vi "Arm Actuator Controller.vi"(8 "error in":errorcluster) -> ()   [LabVIEW 2017]
doc: "This VI executes continuously carrying out the current operation and responding to updates or new operations. It will often contain the timing or control code that is difficult to place directly in TeleOp. This VI generally opens all sensors and motors and isolates the rest of the robot code from knowing how the operations are carried out."
uses:
  <vilib>/Rock Robotics/WPI/Framework/Completion Status.ctl
  Arm Actuator Setpoints.ctl
  Arm Actuator Operations.ctl
  Users/Public/Documents/Cross The Road Electronics/Phoenix-LabVIEW/Motor Controller/Controls/CTRE_Phoenix_MotorControl_ControlMode.ctl
  <vilib>/Rock Robotics/WPI/ThirdParty/Phoenix-LabVIEW/Motor Controller/Controls/CTRE_Phoenix_MotorControl_NeutralMode.ctl
  <vilib>/Rock Robotics/WPI/Solenoid/WPI_SolenoidValue.ctl
  <vilib>/Rock Robotics/WPI/Solenoid/WPI_SolenoidChannel.ctl
  <vilib>/Rock Robotics/WPI/Solenoid/WPI_SolenoidSetEnum.vi
  <vilib>/Rock Robotics/WPI/Solenoid/WPI_SolenoidOpenSingle.vi
  <vilib>/Rock Robotics/Network Tables/NT Write Boolean.vi
panel:
  in  "Interactive Values":T1
  out "Current\nCmd":string
  in  "Buttons":cluster{"Execute Cmd":bool, "Abort Cmd":bool}
  out "Command Timing":cluster{"Start Time (ms)":u32, "Iterations":i32}
  out "Status":T3
  # "Tip: It may be helpful to observe inputs and sensor values.\nYou may also want to display tuning or debugging controls."
  # "Interactive Command: You may fill in the settings for a command\nand schedule it with the Execute button. You can observe and abort\nany command while fine tuning the code for the controller."
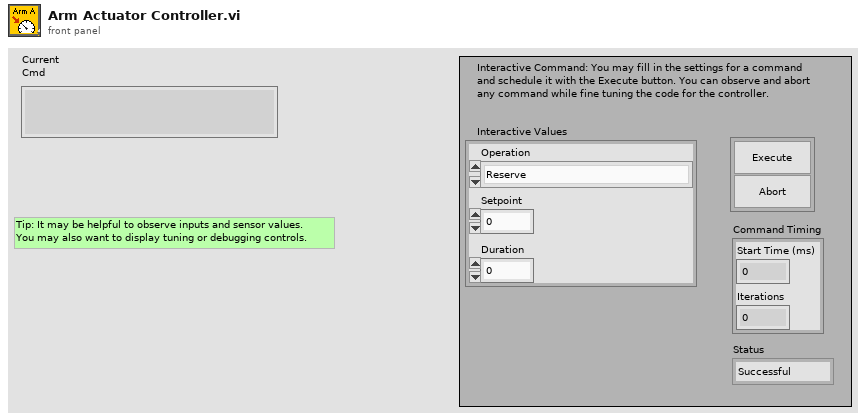
[diagram p1: front panel]
types:
  T1 = typedef "Arm Actuator Setpoints.ctl" = cluster{"Operation":T2, "Setpoint":dbl, "Duration":dbl}
  T2 = typedef "Arm Actuator Operations.ctl" = enum16{"Reserve", "Read Current", "Immediate", "Move Arm", "Claw In", "Claw Out"}
  T3 = typedef "Completion Status.ctl" = enum16{"Successful", "Aborted", "Incomplete"}
  T4 = typedef "WPI_SolenoidChannel.ctl" = enum8{"Solenoid 0", "Solenoid 1", "Solenoid 2", "Solenoid 3", "Solenoid 4", "Solenoid 5", "Solenoid 6", "Solenoid 7", "Invalid"}
  T5 = typedef "WPI_SolenoidValue.ctl" = enum16{"Off", "On", "Forward", "Reverse"}
  T6 = typedef "CTRE_Phoenix_MotorControl_NeutralMode.ctl" = enum8{"EEPROMSetting", "Override to Coast", "Override to Brake"}
  T7 = typedef "CTRE_Phoenix_MotorControl_ControlMode.ctl" = u16
  T8 = typedef "WPI_SolenoidDevRef.ctl" = cluster{"DevStatus":errorcluster, "Pneumatics Control Module":u8, "Forward Solenoid Channel":T4, "Reverse Solenoid Channel":T4}
  T9 = typedef "WPI_MotorControlDeviceRef.ctl" = cluster{"DeviceStatus":errorcluster, "Type":T10, "PWM":cluster{"PWM Channel":T11, "DeadBand":T12}, "CAN":cluster{"Device Number":u8, "SetOutput VI Ref":variant, "GetOutput VI Ref":variant, "Enable VI Ref":variant, "Disable VI Ref":variant, "Data":variant}, "Invert":bool, "DIO PWM":cluster{"PWM \"Enable\" Channel":T11, "DIOChannel":T13, "PWM Rate":dbl}}
  T10 = typedef "WPI_MotorControlType.ctl" = enum16{"PWM", "CAN", "DIO PWM"}
  T11 = typedef "FPGA_DIOPWMChannel.ctl" = enum8{"PWM 0", "PWM 1", "PWM 2", "PWM 3", "PWM 4", "PWM 5", "PWM 6", "PWM 7", "PWM 8", "PWM 9", "PWM MXP 0", "PWM MXP 1", "PWM MXP 2", "PWM MXP 3", "PWM MXP 4", "PWM MXP 5", "PWM MXP 6", "PWM MXP 7", "PWM MXP 8", "PWM MXP 9", "Invalid"}
  T12 = typedef "WPI_PWMDeadband.ctl" = cluster{"Name":string, "maxPositivePwm":i32, "minPositivePwm":i32, "centerPwm":i32, "maxNegativePwm":i32, "minNegativePwm":i32, "angularRange":u16}
  T13 = typedef "FPGA_DIOChannel.ctl" = enum8{"DIO 0", "DIO 1", "DIO 2", "DIO 3", "DIO 4", "DIO 5", "DIO 6", "DIO 7", "DIO 8", "DIO 9", "DIO MXP 0", "DIO MXP 1", "DIO MXP 2", "DIO MXP 3", "DIO MXP 4", "DIO MXP 5", "DIO MXP 6", "DIO MXP 7", "DIO MXP 8", "DIO MXP 9", "DIO MXP 10", "DIO MXP 11", "DIO MXP 12", "DIO MXP 13", "DIO MXP 14", "DIO MXP 15", "SPI Port CS1", "SPI Port CS2", "SPI Port CS3", "SPI Port MISO", "SPI Port MOSI", "Invalid"}
  T14 = typedef "Command Status Info.ctl" = cluster{"Name":string, "Status":T3, "notifier out":T15}
  T15 = typedef "Completion Notifier.ctl" = refnum<notifier>
  T16 = cluster{"Current Command":T1, "Command Timing":cluster{"Start Time (ms)":u32, "Iterations":i32}, "Command Arguments":cluster{"Command Info":T14, "Description":string, "Default Command":T1, "queue out":refnum<queue>, "Subsystem Name":string}}
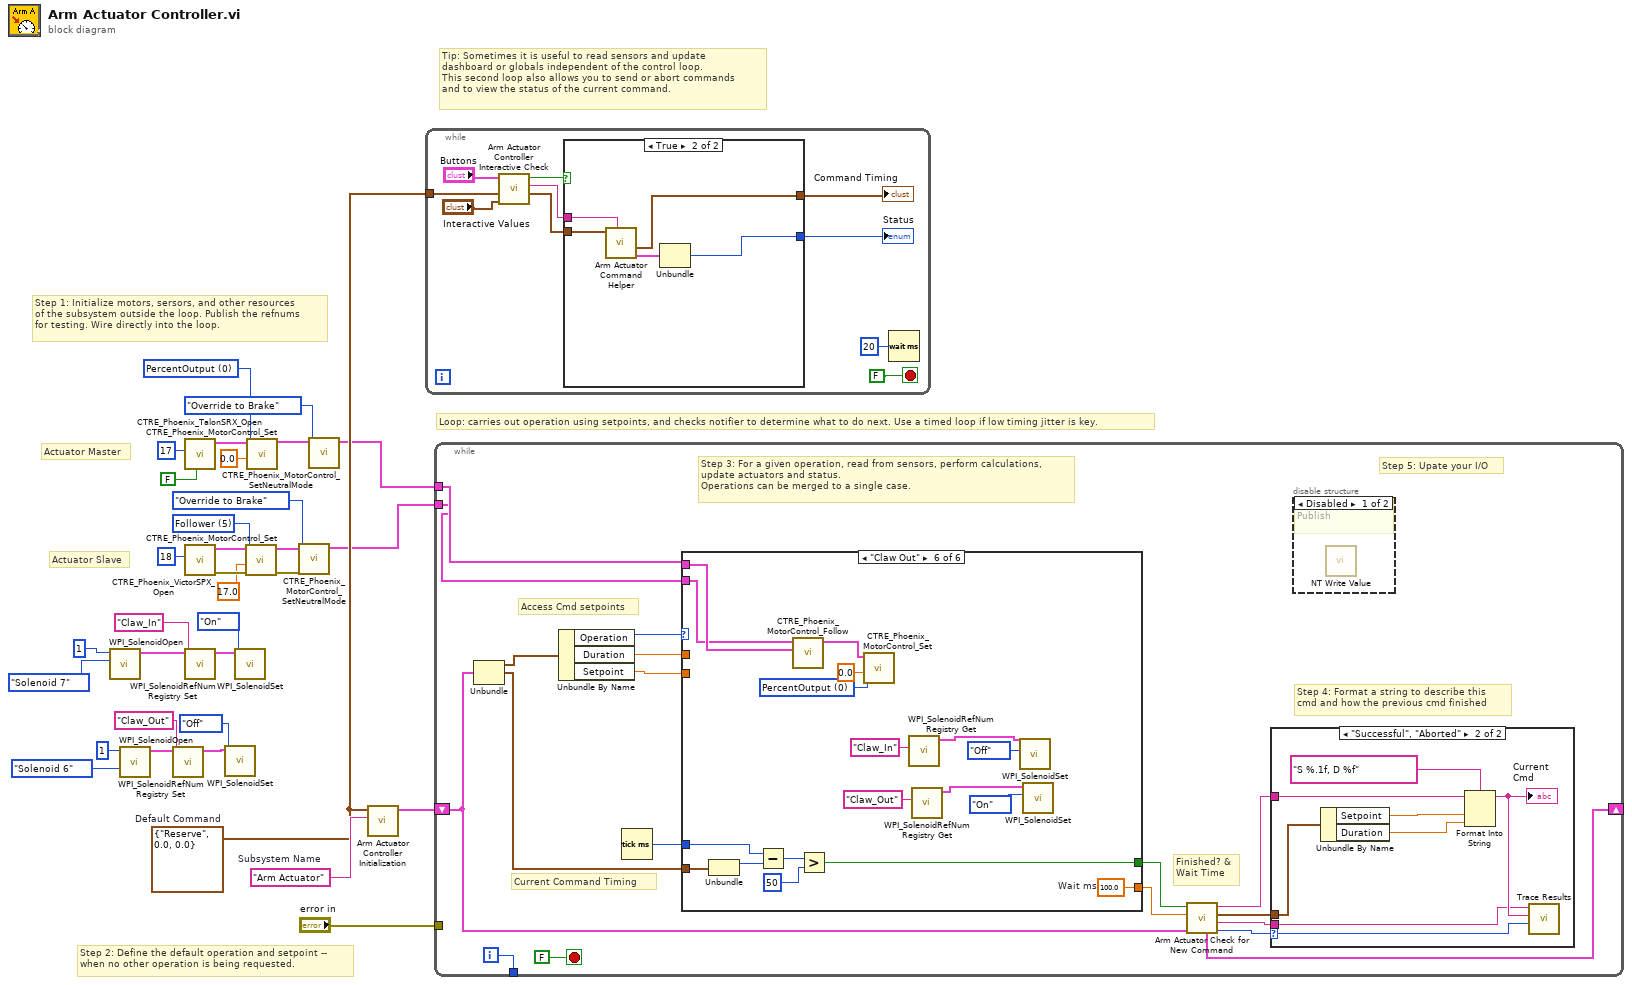
[diagram p0: block diagram]
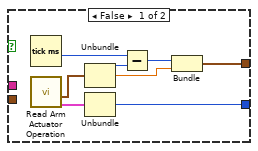
[diagram p2: hidden frame]
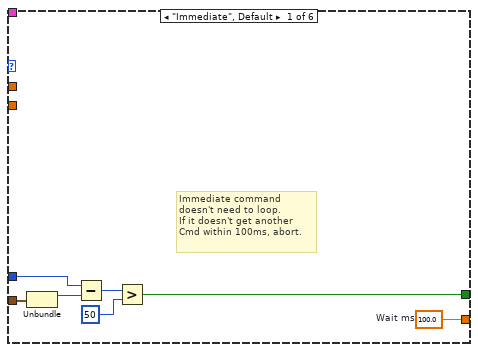
[diagram p5: hidden frame]
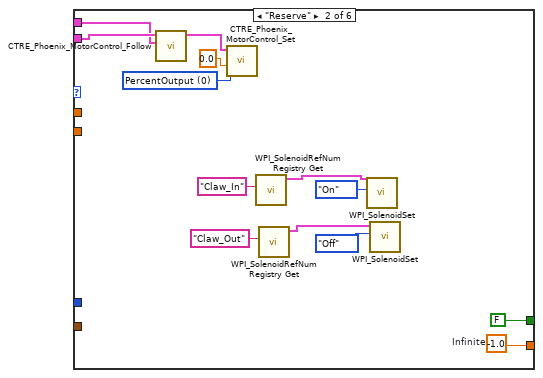
[diagram p6: hidden frame]
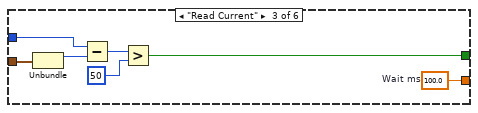
[diagram p7: hidden frame]
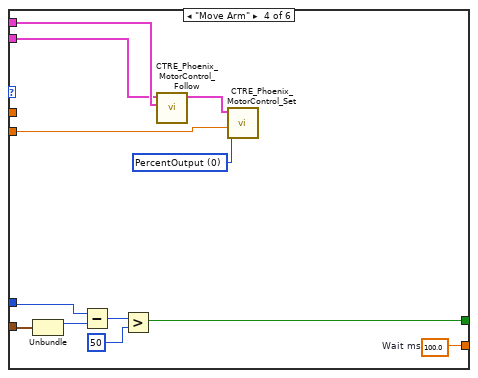
[diagram p8: hidden frame]
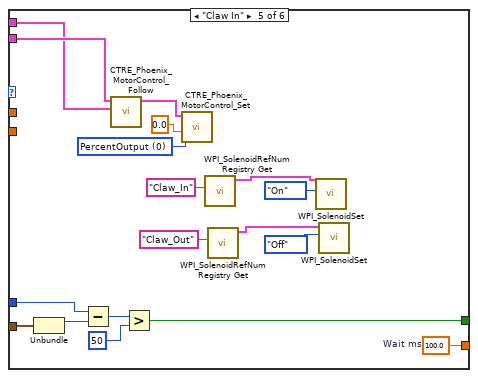
[diagram p9: hidden frame]
diagram:
  w15 = T7 5 items=["PercentOutput"=0, "Position"=1, "Velocity"=2, "Current"=3, "Follower"=5, "MotionProfile"=6, "MotionMagic"=7, "MotionMagicArc"=8, "MotionProfileArc"=10, "Disabled"=15] ("Control Mode")
  w22 = T7 0 items=["PercentOutput"=0, "Position"=1, "Velocity"=2, "Current"=3, "Follower"=5, "MotionProfile"=6, "MotionMagic"=7, "MotionMagicArc"=8, "MotionProfileArc"=10, "Disabled"=15] ("Control Mode")
  w30 = T1 {"Operation"=enum."Reserve", "Setpoint"=0.0, "Duration"=0.0}  # Default Command
  w31 = "Arm Actuator"  # Subsystem Name
  # "Actuator Slave"
  # "Actuator Master"
  # "Tip: Sometimes it is useful to read sensors and update\ndashboard or globals independent of the control loop.\nThis second loop also allows you to send or abort commands\nand to view the status of the current command."
  # "Step 2: Define the default operation and setpoint --\nwhen no other operation is being requested."
  # "Step 1: Initialize motors, sersors, and other resources\nof the subsystem outside the loop. Publish the refnums\nfor testing. Wire directly into the loop."
  # "Loop: carries out operation using setpoints, and checks notifier to determine what to do next. Use a timed loop if low timing jitter is key."
  n1 = call-poly <vilib>:"WPI_SolenoidOpen.vi"("Solenoid Channel"=WPI_SolenoidChannel."Solenoid 7", "Pneumatics Control Module (0)"=u8 1) -> ("SolenoidDevRef"=w29:T8)  [unwired: 8 in, 1 out]
  n2 = call-poly <vilib>:"WPI_SolenoidOpen.vi"("Solenoid Channel"=WPI_SolenoidChannel."Solenoid 6", "Pneumatics Control Module (0)"=u8 1) -> ("SolenoidDevRef"=w27:T8)  [unwired: 8 in, 1 out]
  n3 = call <vilib>:"WPI_SolenoidRefNum Registry Set.vi"("refnum name"="Claw_Out", "SolenoidDevRef"=w27) -> ("SolenoidDevRef"=w8:T8)  [unwired: 8 in, 1 out]
  n4 = call <vilib>:"CTRE_Phoenix_TalonSRX_Open.vi"("Invert"=FALSE, "Device Number"=u8 17) -> ("CAN Talon SRX Ref"=w23:T9)  [unwired: 8 in, 1 out]
  n5 = call <vilib>:"CTRE_Phoenix_VictorSPX_Open.vi"("Device Number"=u8 18) -> ("error out"=w17:errorcluster, "CAN Talon SRX Ref"=w16:T9)  [unwired: 9 in]
  n6 = call <vilib>:"WPI_SolenoidRefNum Registry Set.vi"("refnum name"="Claw_In", "SolenoidDevRef"=w29) -> ("SolenoidDevRef"=w6:T8)  [unwired: 8 in, 1 out]
  n7 = call-poly <vilib>:"WPI_SolenoidSet.vi"("Value"=WPI_SolenoidValue."Off", "SolenoidDevRef"=w8) -> ()  [unwired: 8 in, 2 out]
  n8 = call-poly <vilib>:"WPI_SolenoidSet.vi"("Value"=WPI_SolenoidValue."On", "SolenoidDevRef"=w6) -> ()  [unwired: 8 in, 2 out]
  n9 = call <vilib>:"CTRE_Phoenix_MotorControl_Set.vi"("error in (no error)"=w17, "Output"=17.0, "Control Mode"=w15, "PhoenixMotorControlDevRef"=w16) -> ("error out"=w13:errorcluster, "PhoenixMotorControlDevRef"=w12:T9)  [unwired: 6 in]
  n10 = call <vilib>:"CTRE_Phoenix_MotorControl_Set.vi"("Output"=0.0, "Control Mode"=w22, "PhoenixMotorControlDevRef"=w23) -> ("PhoenixMotorControlDevRef"=w20:T9)  [unwired: 7 in, 1 out]
  n11 = call <vilib>:"CTRE_Phoenix_MotorControl_SetNeutralMode.vi"("error in (no error)"=w13, "Motor Control Neutral Mode"=CTRE_Phoenix_MotorControl_NeutralMode."Override to Brake", "PhoenixMotorControlDevRef"=w12) -> ("PhoenixMotorControlDevRef"=w9:T9)  [unwired: 7 in, 1 out]
  n12 = call <vilib>:"CTRE_Phoenix_MotorControl_SetNeutralMode.vi"("Motor Control Neutral Mode"=CTRE_Phoenix_MotorControl_NeutralMode."Override to Brake", "PhoenixMotorControlDevRef"=w20) -> ("PhoenixMotorControlDevRef"=w10:T9)  [unwired: 8 in, 1 out]
  n13 = call "Arm Actuator Controller Initialization.vi"("Subsystem Name"=w31, "Default Command"=w30) -> ("Current Command"=w32:T16)  [unwired: 9 in]
  n14 = while {
    tunnel: w30 -> [w40]
    stop <- FALSE stop-if-true
    n15 = call "Arm Actuator Controller Interactive Check.vi"("Interactive Command in"="Interactive Values", "Default Command"=w40, "Buttons"="Buttons") -> ("Interactive Command out"=w37:T1, "Trace String"=w38:string, "Schedule"=w39:bool)  [unwired: 6 in]
    n16 = case shown="True" w39 {
      tunnel: [w51 w56] -> w36
      tunnel: w37 -> [_ w54]
      tunnel: [w47 w52] -> w35
      tunnel: w38 -> [_ w55]
      frame False {
        n17 = Tick Count (ms)() -> (millisecond timer value=w46:u32)
        n18 = call "Read Arm Actuator Operation.vi"() -> ("Command Info"=w44:T14, "SubSystem Data"=w45:T1)  [unwired: 9 in, 1 out]
        n19 = Unbundle(w45) -> ("Operation"=w50:T2, "Setpoint"=w48:dbl)  [unwired: 1 out]
        n20 = Unbundle(w44) -> ("Status"=w51:T3)  [unwired: 2 out]
        n21 = Subtract(x=w46, y=w50) -> (x-y=w49:u32)
        n22 = Bundle(w49, "Setpoint"=w48) -> (w47:cluster{u32, "Setpoint":dbl})  [unwired: 1 in]
      }
      frame True {
        n23 = call "Arm Actuator Command Helper.vi"("Description"=w55, "SubSystem Data"=w54) -> ("Command Info Out"=w53:T14, "Command Timing"=w52:cluster{"Start Time (ms)":u32, "Iterations":i32})  [unwired: 7 in, 1 out]
        n24 = Unbundle(w53) -> ("Status"=w56:T3)  [unwired: 2 out]
      }
    }
    "Status" <- w36
    "Command Timing" <- w35
    n25 = Wait (ms)(milliseconds to wait=u32 20) -> ()  [unwired: 1 out]
  }
  n26 = while {
    shift-right: [w66] -> _
    shift-left: w32 -> [w59]
    tunnel: [w73] -> _
    tunnel: "error in" -> [_]
    tunnel: w10 -> [w58]
    tunnel: w9 -> [w57]
    i -> [w73]
    stop <- FALSE stop-if-true
    # "Step 5: Upate your I/O"
    # "Step 4: Format a string to describe this\ncmd and how the previous cmd finished"
    # "Current Command Timing"
    # "Access Cmd setpoints"
    # "Finished? &\nWait Time"
    # "Step 3: For a given operation, read from sensors, perform calculations,\nupdate actuators and status.\nOperations can be merged to a single case."
    n27 = Unbundle(w59) -> ("Current Command"=w72:T1, "Command Timing"=w68:cluster{"Start Time (ms)":u32, "Iterations":i32})  [unwired: 1 out]
    n28 = Unbundle By Name(w72) -> ("Operation"=w71:T2, "Duration"=w70:dbl, "Setpoint"=w67:dbl)
    n29 = Tick Count (ms)() -> (millisecond timer value=w69:u32)
    n30 = case shown="\"Claw Out\"" w71 {
      tunnel: [w89 w102 w104 w116 w133 w152] -> w64
      tunnel: [w83 FALSE ("ignore previous (F)") w105 w115 w134 w151] -> w65
      tunnel: w68 -> [w85 _ w103 w118 w135 w153]
      tunnel: w70 -> [_ _ _ _ _ _]
      tunnel: w69 -> [w84 _ w106 w117 w136 w154]
      tunnel: w67 -> [_ _ _ w112 _ _]
      tunnel: w58 -> [_ w99 _ w111 w128 w147]
      tunnel: w57 -> [_ w100 _ w110 w129 w146]
      frame "Immediate", Default {
        w89 = 100.0  # Wait ms
        # "Immediate command\ndoesn't need to loop.\nIf it doesn't get another\nCmd within 100ms, abort."
        n31 = Unbundle(w85) -> ("Start Time (ms)"=w88:u32)  [unwired: 1 out]
        n32 = Subtract(x=w84, y=w88) -> (x-y=w87:u32)
        n33 = Greater?(x=w87, y=u8 50 ("Left Motor")) -> (0:w83:bool)
      }
      frame "Reserve" {
        w96 = T7 0 items=["PercentOutput"=0, "Position"=1, "Velocity"=2, "Current"=3, "Follower"=5, "MotionProfile"=6, "MotionMagic"=7, "MotionMagicArc"=8, "MotionProfileArc"=10, "Disabled"=15] ("Control Mode")
        w102 = -1.0  # Infinite
        n34 = call <vilib>:"CTRE_Phoenix_MotorControl_Follow.vi"("Master Controller to Follow"=w99, "PhoenixMotorControlDevRef"=w100) -> ("PhoenixMotorControlDevRef"=w98:T9)  [unwired: 8 in, 1 out]
        n35 = call <vilib>:"CTRE_Phoenix_MotorControl_Set.vi"("Output"=0.0, "Control Mode"=w96, "PhoenixMotorControlDevRef"=w98) -> ()  [unwired: 7 in, 2 out]
        n36 = call <vilib>:"WPI_SolenoidRefNum Registry Get.vi"("refnum name"="Claw_In") -> ("SolenoidDevRef"=w92:T8)  [unwired: 9 in, 1 out]
        n37 = call <vilib>:"WPI_SolenoidRefNum Registry Get.vi"("refnum name"="Claw_Out") -> ("SolenoidDevRef"=w90:T8)  [unwired: 9 in, 1 out]
        n38 = call-poly <vilib>:"WPI_SolenoidSet.vi"("Value"=WPI_SolenoidValue."On", "SolenoidDevRef"=w92) -> ()  [unwired: 8 in, 2 out]
        n39 = call-poly <vilib>:"WPI_SolenoidSet.vi"("Value"=WPI_SolenoidValue."Off", "SolenoidDevRef"=w90) -> ()  [unwired: 8 in, 2 out]
      }
      frame "Read Current" {
        w104 = 100.0  # Wait ms
        n40 = Unbundle(w103) -> ("Start Time (ms)"=w109:u32)  [unwired: 1 out]
        n41 = Subtract(x=w106, y=w109) -> (x-y=w108:u32)
        n42 = Greater?(x=w108, y=u8 50 ("Left Motor")) -> (0:w105:bool)
      }
      frame "Move Arm" {
        w113 = T7 0 items=["PercentOutput"=0, "Position"=1, "Velocity"=2, "Current"=3, "Follower"=5, "MotionProfile"=6, "MotionMagic"=7, "MotionMagicArc"=8, "MotionProfileArc"=10, "Disabled"=15] ("Control Mode")
        w116 = 100.0  # Wait ms
        n43 = Unbundle(w118) -> ("Start Time (ms)"=w120:u32)  [unwired: 1 out]
        n44 = Subtract(x=w117, y=w120) -> (x-y=w121:u32)
        n45 = Greater?(x=w121, y=u8 50 ("Left Motor")) -> (0:w115:bool)
        n46 = call <vilib>:"CTRE_Phoenix_MotorControl_Follow.vi"("Master Controller to Follow"=w111, "PhoenixMotorControlDevRef"=w110) -> ("PhoenixMotorControlDevRef"=w114:T9)  [unwired: 8 in, 1 out]
        n47 = call <vilib>:"CTRE_Phoenix_MotorControl_Set.vi"("Output"=w112, "Control Mode"=w113, "PhoenixMotorControlDevRef"=w114) -> ()  [unwired: 7 in, 2 out]
      }
      frame "Claw In" {
        w130 = T7 0 items=["PercentOutput"=0, "Position"=1, "Velocity"=2, "Current"=3, "Follower"=5, "MotionProfile"=6, "MotionMagic"=7, "MotionMagicArc"=8, "MotionProfileArc"=10, "Disabled"=15] ("Control Mode")
        w133 = 100.0  # Wait ms
        n48 = Unbundle(w135) -> ("Start Time (ms)"=w139:u32)  [unwired: 1 out]
        n49 = Subtract(x=w136, y=w139) -> (x-y=w138:u32)
        n50 = call <vilib>:"CTRE_Phoenix_MotorControl_Follow.vi"("Master Controller to Follow"=w128, "PhoenixMotorControlDevRef"=w129) -> ("PhoenixMotorControlDevRef"=w132:T9)  [unwired: 8 in, 1 out]
        n51 = Greater?(x=w138, y=u8 50 ("Left Motor")) -> (0:w134:bool)
        n52 = call <vilib>:"CTRE_Phoenix_MotorControl_Set.vi"("Output"=0.0, "Control Mode"=w130, "PhoenixMotorControlDevRef"=w132) -> ()  [unwired: 7 in, 2 out]
        n53 = call <vilib>:"WPI_SolenoidRefNum Registry Get.vi"("refnum name"="Claw_In") -> ("SolenoidDevRef"=w124:T8)  [unwired: 9 in, 1 out]
        n54 = call <vilib>:"WPI_SolenoidRefNum Registry Get.vi"("refnum name"="Claw_Out") -> ("SolenoidDevRef"=w122:T8)  [unwired: 9 in, 1 out]
        n55 = call-poly <vilib>:"WPI_SolenoidSet.vi"("Value"=WPI_SolenoidValue."On", "SolenoidDevRef"=w124) -> ()  [unwired: 8 in, 2 out]
        n56 = call-poly <vilib>:"WPI_SolenoidSet.vi"("Value"=WPI_SolenoidValue."Off", "SolenoidDevRef"=w122) -> ()  [unwired: 8 in, 2 out]
      }
      frame "Claw Out" {
        w148 = T7 0 items=["PercentOutput"=0, "Position"=1, "Velocity"=2, "Current"=3, "Follower"=5, "MotionProfile"=6, "MotionMagic"=7, "MotionMagicArc"=8, "MotionProfileArc"=10, "Disabled"=15] ("Control Mode")
        w152 = 100.0  # Wait ms
        n57 = Unbundle(w153) -> ("Start Time (ms)"=w156:u32)  [unwired: 1 out]
        n58 = Subtract(x=w154, y=w156) -> (x-y=w157:u32)
        n59 = call <vilib>:"CTRE_Phoenix_MotorControl_Follow.vi"("Master Controller to Follow"=w147, "PhoenixMotorControlDevRef"=w146) -> ("PhoenixMotorControlDevRef"=w150:T9)  [unwired: 8 in, 1 out]
        n60 = Greater?(x=w157, y=u8 50 ("Left Motor")) -> (0:w151:bool)
        n61 = call <vilib>:"CTRE_Phoenix_MotorControl_Set.vi"("Output"=0.0, "Control Mode"=w148, "PhoenixMotorControlDevRef"=w150) -> ()  [unwired: 7 in, 2 out]
        n62 = call <vilib>:"WPI_SolenoidRefNum Registry Get.vi"("refnum name"="Claw_In") -> ("SolenoidDevRef"=w142:T8)  [unwired: 9 in, 1 out]
        n63 = call <vilib>:"WPI_SolenoidRefNum Registry Get.vi"("refnum name"="Claw_Out") -> ("SolenoidDevRef"=w140:T8)  [unwired: 9 in, 1 out]
        n64 = call-poly <vilib>:"WPI_SolenoidSet.vi"("Value"=WPI_SolenoidValue."Off", "SolenoidDevRef"=w142) -> ()  [unwired: 8 in, 2 out]
        n65 = call-poly <vilib>:"WPI_SolenoidSet.vi"("Value"=WPI_SolenoidValue."On", "SolenoidDevRef"=w140) -> ()  [unwired: 8 in, 2 out]
      }
    }
    n66 = call "Arm Actuator Check for New Command.vi"("Current Command"=w59, "Wait time (ms)"=w64, "Finished?"=w65) -> ("Completion"=w60:T3, "Subsystem Name"=w61:string, "Current Command"=w62:T1, "Initial Trace String"=w63:string, "NextCommand"=w66:T16)  [unwired: 4 in]
    n67 = case shown="\"Successful\", \"Aborted\"" w60 {
      selector: w60 -> [_ w82]
      tunnel: w63 -> [_ w78]
      tunnel: w62 -> [_ w79]
      tunnel: w61 -> [_ w75]
      frame "Incomplete", Default {
        # "Continuing current command"
      }
      frame "Successful", "Aborted" {
        # "Report and setup for next command"
        n68 = Unbundle By Name(w79) -> ("Setpoint"=w81:dbl, "Duration"=w76:dbl)
        n69 = Format Into String(format string="S %.1f, D %f", initial string=w78, w81, w76) -> (resulting string=w77:string)  [unwired: 1 in, 1 out]
        "Current\nCmd" <- w77
        n70 = call <vilib>:"Trace Results.vi"("Status of previous command"=w82, "Description"=w77, "Subsystem"=w75) -> ()  [unwired: 9 in]
      }
    }
    n71 = disable-structure shown="Disabled" {
      frame Disabled {
        # "Publish"
        n72 = call-poly <vilib>:"NT Write Value.vi"() -> ()  [unwired: 11 in, 1 out]
      }
      frame Enabled {
      }
    }
  }
